vi "Remove Block Diagram Code from Method VI.vi"(8 "error in (no error)":errorcluster, 11 "Method VI Path":path) -> (0 "error out":errorcluster)   [LabVIEW 2016, in "SLL Scripting.lvlib" / "SLL Class DVR API Generator.lvlib"]
uses:
  SLL Class DVR API Generator.lvlib
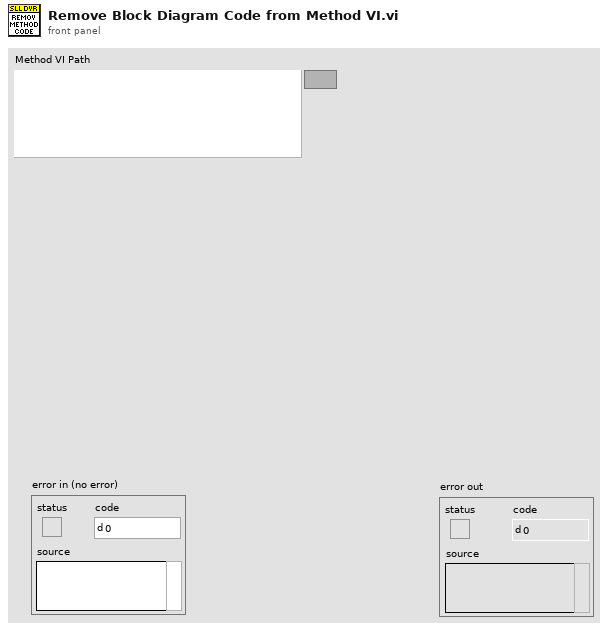
[diagram p1: front panel]
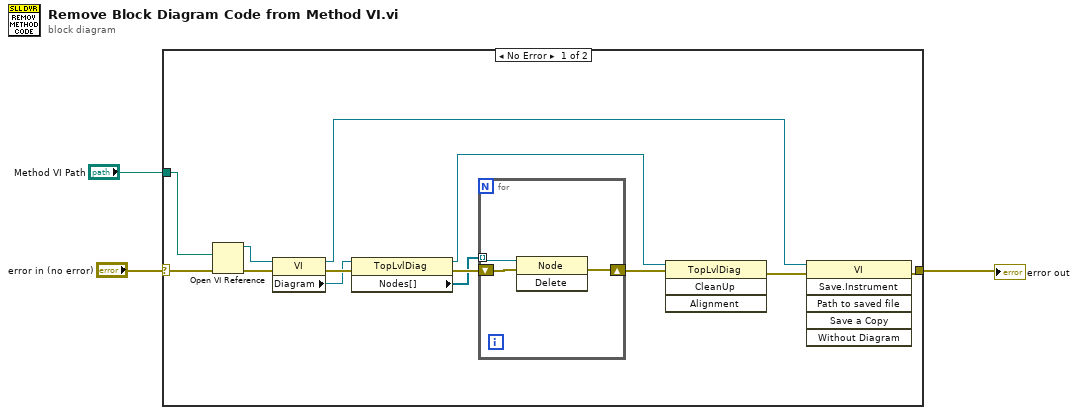
[diagram p0: block diagram]
diagram:
  n1 = case shown="No Error" "error in (no error)" {
    selector: "error in (no error)" -> [w16 w20]
    tunnel: [w6 w20] -> w2
    tunnel: "Method VI Path" -> [w14 _]
    frame No Error {
      n2 = Open VI Reference(vi path=w14, error in (no error)=w16) -> (vi reference=w11:refnum<vi>, error out=w15:errorcluster)  [unwired: 4 in]
      n3 = property class="VI"(reference=w11, error in=w15) -> (reference out=w4:refnum<vi>, error out=w13:errorcluster, "Diagram"=w12:refnum<vi>)
      n4 = property class="TopLvlDiag"(reference=w12, error in=w13) -> (reference out=w7:refnum<vi>, error out=w10:errorcluster, "Nodes[]"=w9:refnum<vi>[])
      n5 = for {
        tunnel: w9 -> [w18] mode=indexing
        shift-right: [w17] -> w8
        shift-left: w10 -> [w19]
        n6 = invoke class="Node" method="Delete"(reference=w18, error in=w19) -> (error out=w17:errorcluster)  [unwired: 1 in, 2 out]
      }
      n7 = invoke class="TopLvlDiag" method="CleanUp"(reference=w7, error in=w8) -> (error out=w5:errorcluster)  [unwired: 2 in, 3 out]
      n8 = invoke class="VI" method="Save.Instrument"(reference=w4, error in=w5) -> (error out=w6:errorcluster)  [unwired: 4 in, 5 out]
    }
    frame Error {
    }
  }
  "error out" <- w2
